vi "Rate Selective Filter.vi"(4 "Hyster":dbl=0.3, 5 "Rate Thresh":dbl=25.0 step=0.001, 6 "hi limit":dbl=50.0, 7 "lo limit":dbl, 8 "Time":dbl, 9 "Distance":dbl) -> (0 "Mode":bool, 1 "OOR":bool, 3 "Filtered":dbl)   [LabVIEW 2013]
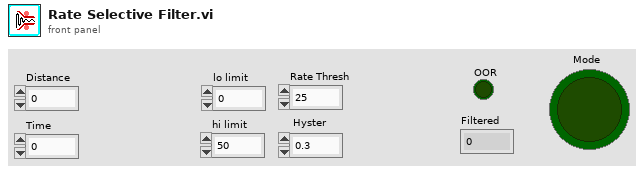
[diagram p1: front panel]
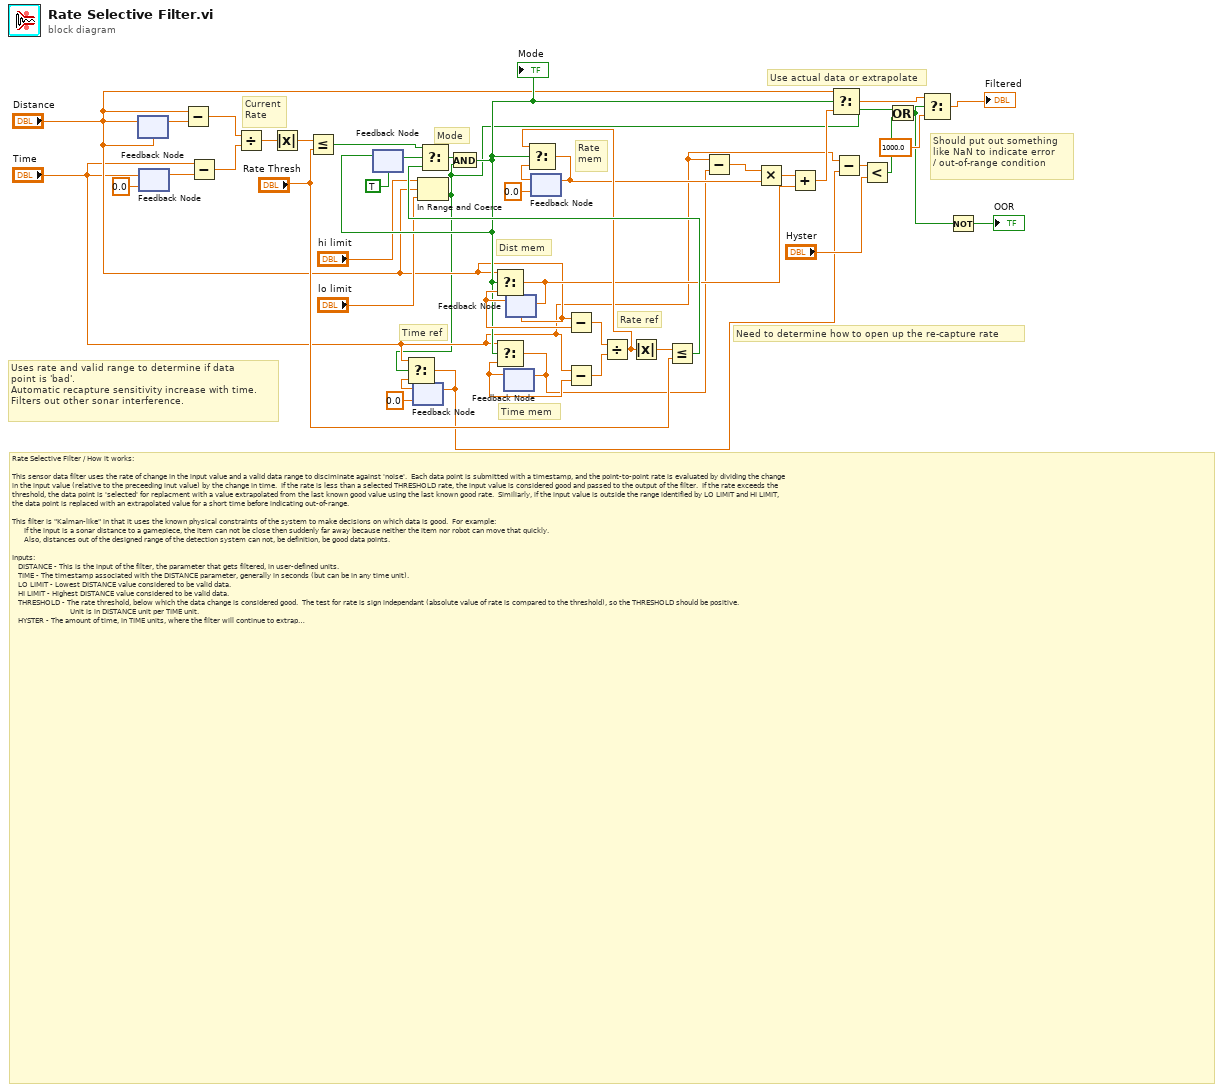
[diagram p0: block diagram]
diagram:
  # "Rate Selective Filter / How it works:\n\nThis sensor data filter uses the rate of change in the input value and a valid data range to disciminate against 'noise'.  Each data point is submitted with a timestamp, and the point-to-point rate is evaluated by dividing the change\nin the input value (relative to the preceeding inut value) by the change in time.  If the rate is less than a selected THRESHOLD rate, the input value is considered good and passed to the output of the filter.  If the rate exceeds the\nthreshold, the data point is 'selected' for replacment with a value extrapolated from the last known good value using the last known good rate.  Similiarly, if the input value is outside the range identified by LO LIMIT and HI LIMIT,\nthe data point is replaced with an extrapolated value for a short time before indicating out-of-range.\n\nThis filter is \"Kalman-like\" in that it uses the known physical constraints of the system to make decisions on which data is good.  For example:\n      If the input is a sonar distance to a gamepiece, the item can not be close then suddenly far away because neither the item nor robot can move that quickly.\n      Also, distances out of the designed range of the detection system can not, be definition, be good data points.\n\nInputs:\n   DISTANCE - This is the input of the filter, the parameter that gets filtered, in user-defined units.\n   TIME - The timestamp associated with the DISTANCE parameter, generally in seconds (but can be in any time unit).\n   LO LIMIT - Lowest DISTANCE value considered to be valid data.\n   HI LIMIT - Highest DISTANCE value considered to be valid data.\n   THRESHOLD - The rate threshold, below which the data change is considered good.  The test for rate is sign independant (absolute value of rate is compared to the threshold), so the THRESHOLD should be positive.\n                             Unit is in DISTANCE unit per TIME unit.\n   HYSTER - The amount of time, in TIME units, where the filter will continue to extrapolate values when the DISTANCE parameter has gone out-of-range.  This provides a degree of hystereis allowing momentary data excursions to\n                     be smoothed before reporting OOR.\nOutputs:\n   FILTERED - Output of filter, depending on rate and range, will either be equal to the input DISTANCE, or extrapolated, or \"0\" (indicating out-of-range).\n   OOR - Boolean Out-of-Range indicator.  True when input DISTANCE is below LO LIMIT or above HI LIMIT.  False when within or equal to defined limits.\n   MODE - Boolean indication of filter mode for corresponding data point.  True when input DISTANCE passes rate and range test and FILTERED value is DISTANCE value.  False when tests fail and FILTERED is an extrapolated value.\n\nInitial Conditions:\n   Rate - The initial rate calculation for the first data point will be zero.\n   Mode - The initial mode of the filter is to consider the inital data point good, as long as it is in range.\n   \nSetting Guidance:\n   Set LO and HI LIMITS to specify the range of acceptable/meaningful DISTANCE values.\n   Set THRESHOLD to the highest expected rate of change believed to be possible for meaningful DISTANCE values given the physical system.  The filter is tolerant of somewhat lower settings, as the effect will only be to replace\n         otherwise 'good' data with very slightly different extrapolated values.  Severe lowering of THRESHOLD will result in over extrapolation and degraded responsiveness to meaningful input data.\n   Set HYSTER to the amount of time that momentary/spurious out-of-range data typically takes to return to normal.  Tradeoff is that longer times delay the reporting of sustained out-of-range conditions.\n\nBehavior:\n   This filter is 'Rate Priority', in the sense that it favors a situation where DISTANCE is changing, rather than static situations.  If a data point is determined to be 'bad', it creates replacement data by extrapolating using the previous\n    rate of change.  In a changing situation, this is more likely to maintain the fidelity of the measurand, since the change rate will likely dominate the predictability of next data point.  This is why the replacement point was not\n    chosen to be a simple repeat of the preceeding data point.  The tradeoff is that this approach can create artificial rate projections purely from sensor noise in static situations, which can lead to poor results.  The rate\n    extrapolation approach is chosen since this filter was designed solely for use where the input is changing (control while closing a sonar distance).\n\n   The RoboBees Team 836"
  # "Use actual data or extrapolate"
  # "Rate ref"
  # "Current\nRate"
  # "Time ref"
  # "Uses rate and valid range to determine if data\npoint is 'bad'.\nAutomatic recapture sensitivity increase with time.\nFilters out other sonar interference."
  # "Need to determine how to open up the re-capture rate"
  # "Should put out something\nlike NaN to indicate error\n/ out-of-range condition"
  # "Rate\nmem"
  # "Mode"
  # "Time mem"
  # "Dist mem"
  n1 = feedback #1("Distance") -> (w40:dbl)
  n2 = feedback-in #1("Distance") -> ()
  n3 = feedback #2(0.0) -> (w39:dbl)
  n4 = feedback-in #2("Time") -> ()
  n5 = Subtract(x="Distance", y=w40) -> (x-y=w44:dbl)
  n6 = Subtract(x="Time", y=w39) -> (x-y=w43:dbl)
  n7 = Divide(x=w44, y=w43) -> (x/y=w2:dbl)
  n8 = Absolute Value(x=w2) -> (abs(x)=w38:dbl)
  n9 = Less Or Equal?(x=w38, y="Rate Thresh") -> (x <= y?=w22:bool)
  n10 = feedback #3(TRUE) -> (w41:bool)
  n11 = feedback #4(0.0) -> (w15:dbl)
  n12 = In Range and Coerce(upper limit="hi limit", x="Distance", lower limit="lo limit") -> (In Range?=w1:bool)  [unwired: 1 out]
  n13 = Select(t="Time", s=w1, f=w15) -> (s? t:f=w9:dbl)
  n14 = feedback-in #4(w9) -> ()
  n15 = feedback #5() -> (w34:dbl)  [unwired: 1 in]
  n16 = feedback #6("Distance") -> (w35:dbl)
  n17 = feedback #7(0.0) -> (w30:dbl)
  n18 = Subtract(x="Distance", y=w35) -> (x-y=w36:dbl)
  n19 = Subtract(x="Time", y=w34) -> (x-y=w37:dbl)
  n20 = Divide(x=w36, y=w37) -> (x/y=w25:dbl)
  n21 = Absolute Value(x=w25) -> (abs(x)=w33:dbl)
  n22 = Less Or Equal?(x=w33, y="Rate Thresh") -> (x <= y?=w31:bool)
  n23 = Select(t=w22, s=w41, f=w31) -> (s? t:f=w18:bool)
  n24 = And(x=w18, y=w1) -> (x .and. y?=w19:bool)
  "Mode" <- w19
  n25 = feedback-in #3(w19) -> ()
  n26 = Select(t="Distance", s=w19, f=w35) -> (s? t:f=w24:dbl)
  n27 = Select(t="Time", s=w19, f=w34) -> (s? t:f=w10:dbl)
  n28 = feedback-in #5(w10) -> ()
  n29 = feedback-in #6(w24) -> ()
  n30 = Select(t=w25, s=w19, f=w30) -> (s? t:f=w23:dbl)
  n31 = feedback-in #7(w23) -> ()
  n32 = Subtract(x="Time", y=w10) -> (x-y=w29:dbl)
  n33 = Multiply(x=w29, y=w23) -> (x*y=w28:dbl)
  n34 = Add(x=w28, y=w24) -> (x+y=w27:dbl)
  n35 = Select(t="Distance", s=w19, f=w27) -> (s? t:f=w13:dbl)
  n36 = Subtract(x="Time", y=w9) -> (x-y=w12:dbl)
  n37 = Less?(x=w12, y="Hyster") -> (x < y?=w8:bool)
  n38 = Or(x=w1, y=w8) -> (x .or. y?=w4:bool)
  n39 = Select(t=w13, s=w4, f=1000.0) -> (s? t:f=→"Filtered":dbl)
  n40 = Not(x=w4) -> (.not. x?=→"OOR":bool)
